vi "toml_api_list_sections.vi"(7 "resolved path":path, 8 "error in (no error)":errorcluster, 11 "vi in":refnum<vi>) -> (0 "error out":errorcluster, 1 "sections":string[](array[string]), 2 "file loaded":bool, 3 "vi out":refnum<vi>)   [LabVIEW 2017]
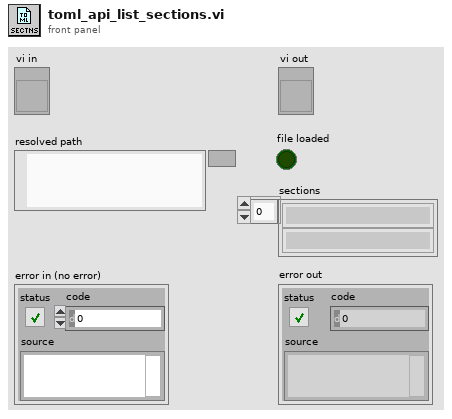
[diagram p1: front panel]
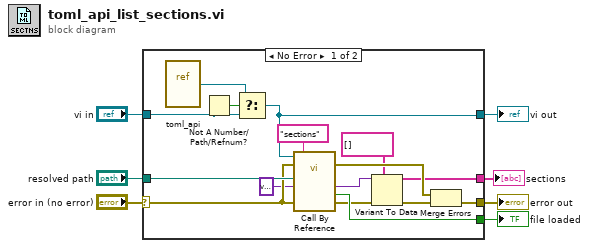
[diagram p0: block diagram]
diagram:
  n1 = case shown="No Error" "error in (no error)" {
    selector: "error in (no error)" -> [w15 w25]
    tunnel: [w23 _] -> w7
    tunnel: "resolved path" -> [w21 _]
    tunnel: [w17 w25] -> w5
    tunnel: "vi in" -> [w14 w24]
    tunnel: [w13 w24] -> w2
    tunnel: [w9 _] -> w1
    frame No Error {
      n2 = vi-ref "toml_api.vi"() -> (w20:refnum<vi>)
      n3 = Not A Number/Path/Refnum?(number/path/refnum=w14) -> (NaN/Path/Refnum?=w19:bool)
      n4 = Select(t=w20, s=w19, f=w14) -> (s? t:f=w13:refnum<vi>)
      n5 = call-by-ref "?"(reference=w13, error in=w15, "cmd"="sections", 8:"error in (no error)"=w15, "data in"=variant, "path in"=w21) -> (error out=w16:errorcluster, 0:"error out"=w22:errorcluster, "return"=w23:bool, "data out"=w11:variant)  [unwired: 4 in, 2 out]
      n6 = Variant To Data(error in=w22, type=string[] [], Variant=w11) -> (data=w9:string[], error out=w12:errorcluster)
      n7 = Merge Errors(w16, w12) -> (w17:errorcluster)
    }
    frame Error {
    }
  }
  "file loaded" <- w7
  "error out" <- w5
  "vi out" <- w2
  "sections" <- w1
